vi "YAG_Control.v6.vi"() -> ()   [LabVIEW 2022 SP3]
uses:
  YAGControl.ctl
panel:
  in  "VISA resource name":refnum<visa-resource-name>="BigSky"
  in  "Cluster":T1={"Lamp mode"=TRUE, "Lamps"=FALSE, "Shutter"=FALSE, "Q-Switch"=FALSE, "Int Rep Rate  "=15.0, "Voltage "=700.0, "Temperature"=39.0, "Quit"=FALSE} {"Int Rep Rate" min=1.0 max=30.0; "Temperature" format="%#.0f"; "Voltage" min=680.0 max=990.0 step=1.0}
  in  "Send":bool
  out "Last Response":string
  in  "Other Command":string="vmo1100"
  # "o"
  # "C"
  # "Hz"
  # "V"
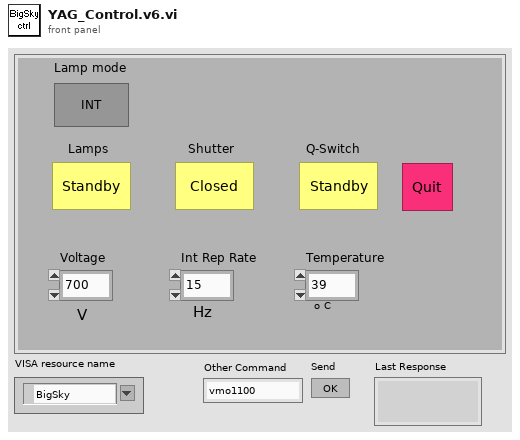
[diagram p1: front panel]
types:
  T1 = typedef "YAGControl.ctl" = cluster{"Lamp mode":bool, "Lamps":bool, "Shutter":bool, "Q-Switch":bool, "Int Rep Rate  ":dbl, "Voltage ":dbl, "Temperature":dbl, "Quit":bool}
  T2 = enum8{"Enabled", "Disabled", "Disabled and Grayed Out"}
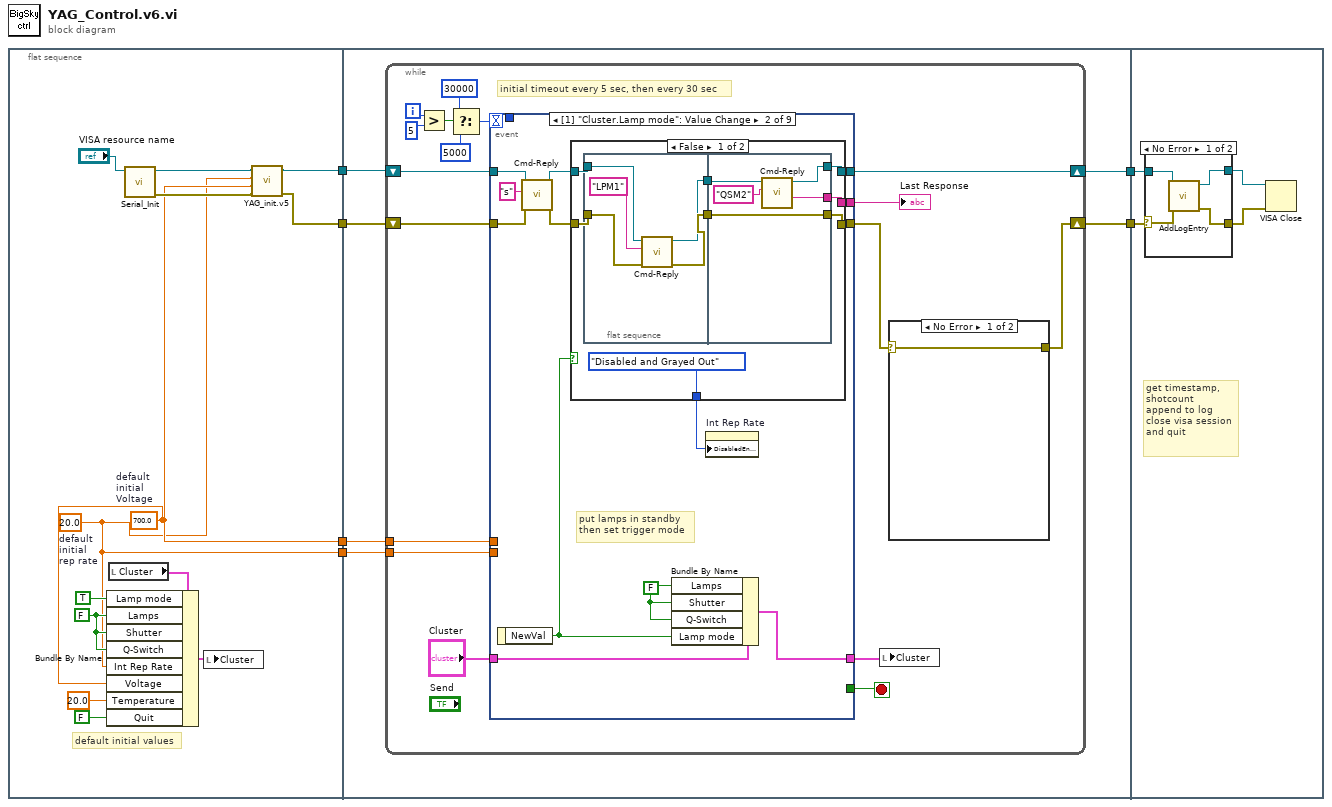
[diagram p0: block diagram]
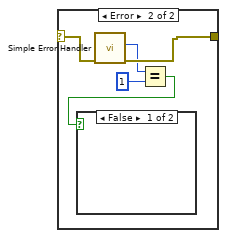
[diagram p2: hidden frame]
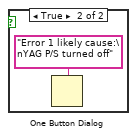
[diagram p3: hidden frame]
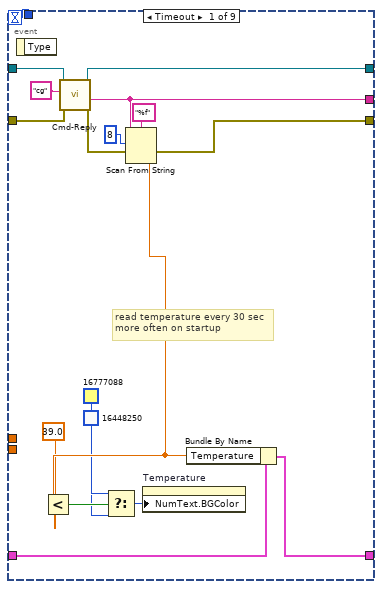
[diagram p4: hidden frame]
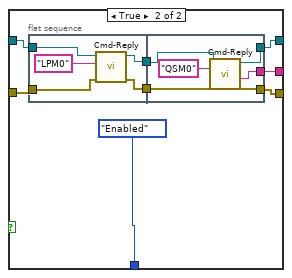
[diagram p5: hidden frame]
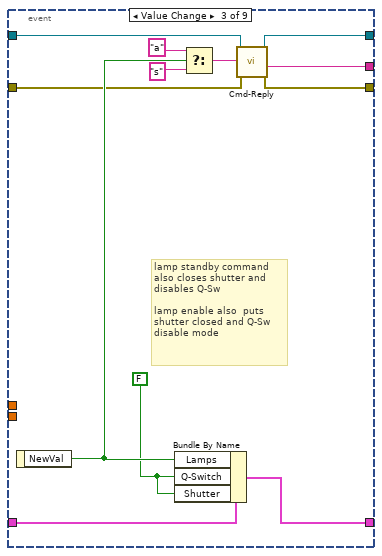
[diagram p6: hidden frame]
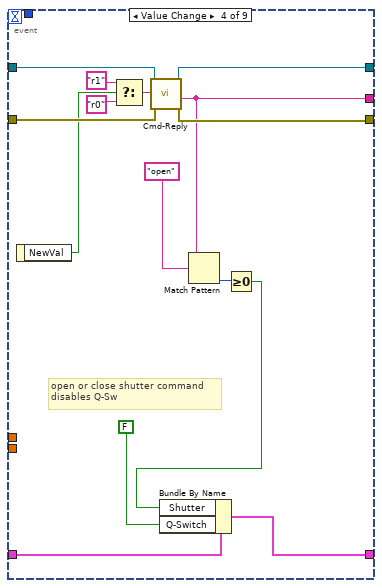
[diagram p7: hidden frame]
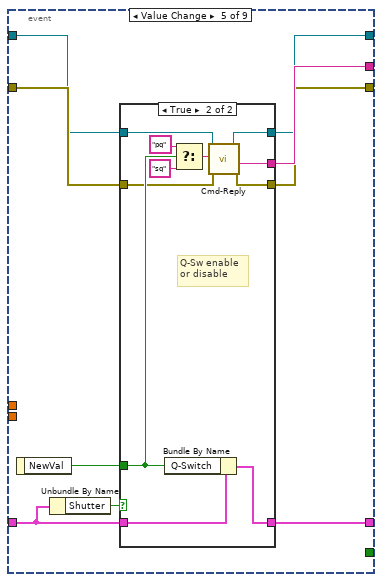
[diagram p8: hidden frame]
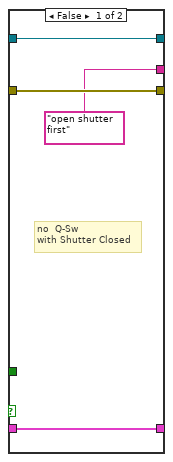
[diagram p9: hidden frame]
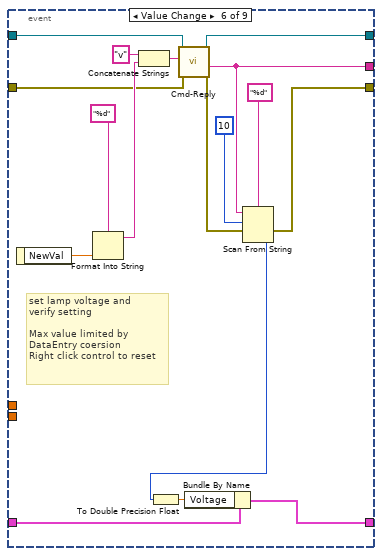
[diagram p10: hidden frame]
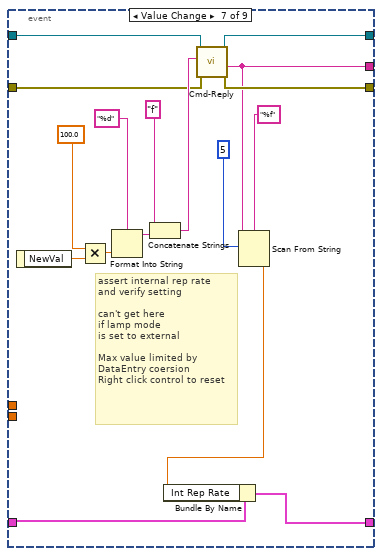
[diagram p11: hidden frame]
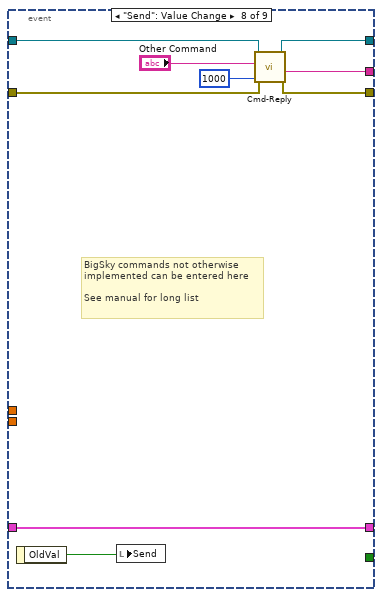
[diagram p12: hidden frame]
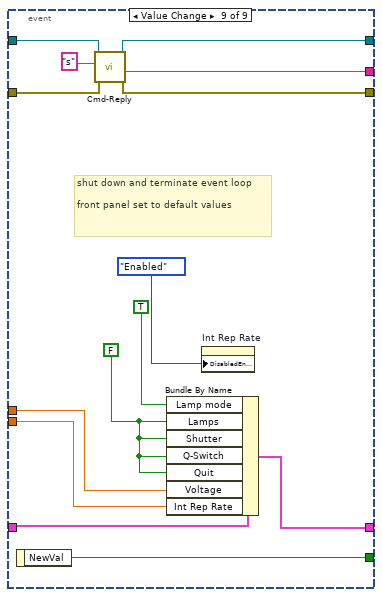
[diagram p13: hidden frame]
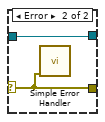
[diagram p14: hidden frame]
diagram:
  n1 = flat-sequence {
    tunnel: [w11] -> w4
    tunnel: [w10] -> w3
    tunnel: [w8] -> w2
    tunnel: [w7] -> w1
    tunnel: [w25] -> w6
    tunnel: [w24] -> w5
    tunnel: w4 -> [w23]
    tunnel: w3 -> [w22]
    tunnel: w2 -> [w21]
    tunnel: w1 -> [w20]
    tunnel: w6 -> [w225]
    tunnel: w5 -> [w228]
    frame #0 {
      w7 = 20.0  # default initial rep rate
      w8 = 700.0  # default  initial Voltage
      w18 = FALSE ("Lamp mode")
      # "default initial values"
      n2 = local read "Cluster"() -> (w13:T1)
      n3 = Bundle By Name(cluster=w13, "Lamp mode"=TRUE, "Lamps"=w18, "Shutter"=w18, "Q-Switch"=w18, "Int Rep Rate"=w7, "Voltage"=w8, "Temperature"=20.0, "Quit"=FALSE) -> (w15:T1)
      n4 = call "Serial_Init.vi"("VISA resource name"="VISA resource name") -> ("error out"=w9:errorcluster, "VISA resource name out"=w12:refnum<visa-resource-name>)  [unwired: 9 in]
      n5 = local write "Cluster"(w15) -> ()
      n6 = call "YAG_init.v5.vi"("error in (no error)"=w9, "initial V"=w8, "initial rep rate"=w7, "VISA Refnum in"=w12) -> ("error out"=w10:errorcluster, "VISA Refnum out"=w11:refnum<visa-resource-name>)  [unwired: 6 in]
    }
    frame #1 {
      n7 = while {
        shift-right: [w36] -> w24
        shift-left: w23 -> [w38]
        shift-right: [w34] -> w25
        shift-left: w22 -> [w37]
        tunnel: w21 -> [w27]
        tunnel: w20 -> [w26]
        i -> [w30]
        stop <- w42 stop-if-true
        # "initial timeout every 5 sec, then every 30 sec"
        n8 = Greater?(x=w30, y=5) -> (0:w28:bool)
        n9 = Select(t=30000, s=w28, f=5000) -> (s? t:f=w33:i32)
        n10 = event shown="[1] \"Cluster.Lamp mode\": Value Change" {
          selector: _ -> [_ _ _ _ _ _ _ _ _]
          dyn-events: _ -> [_ _ _ _ _ _ _ _ _]
          timeout: w33 -> [w51 _ _ _ _ _ _ _ _]
          tunnel: [_ _ _ _ _ _ _ _ w222] -> w42
          tunnel: "Cluster" -> [w67 w80 w128 w143 w150 w168 w200 w210 w224]
          tunnel: [w66 w79 w123 w142 w152 w184 w199 w210 w223] -> w39
          tunnel: [w61 w77 w122 w133 w148 w174 w189 w208 w216] -> w41
          tunnel: w38 -> [w63 w72 w118 w136 w144 w176 w191 w206 w219]
          tunnel: w37 -> [w64 w69 w119 w135 w145 w178 w190 w205 w220]
          tunnel: [w58 w73 w120 w137 w146 w170 w198 w204 w215] -> w35
          tunnel: [w62 w74 w121 w138 w147 w177 w197 w203 w217] -> w36
          tunnel: [w51 _ _ _ _ _ _ _ _] -> _
          tunnel: w27 -> [_ _ _ _ _ _ _ _ w212]
          tunnel: w26 -> [_ _ _ _ _ _ _ _ w211]
          event Timeout {
            # "read temperature every 30 sec\nmore often on startup"
            n11 = event-data() -> ()  [unwired: 1 in, 1 out]
            n12 = call "Cmd-Reply.vi"("error in (no error)"=w64, "cmd"="cg" ("write buffer"), "VISA Refnum in"=w63) -> ("error out"=w59:errorcluster, "reply"=w61:string, "VISA Refnum out"=w62:refnum<visa-resource-name>)  [unwired: 6 in]
            n13 = Scan From String(format string="%f", input string=w61, initial scan location=u32 8, error in=w59) -> (error out=w58:errorcluster, output 1=w57:dbl)  [unwired: 1 in, 2 out]
            n14 = Less?(x=w57, y=39.0) -> (x < y?=w54:bool)
            n15 = Select(t=u32 16777088 ("Color"), s=w54, f=u32 16448250 ("Color")) -> (s? t:f=w55:u32)
            n16 = property on="Temperature" class="DigNum (strict)"("NumText.BGColor"=w55) -> ()  [unwired: 2 in, 2 out]
            n17 = Bundle By Name(cluster=w67, "Temperature"=w57) -> (w66:T1)
          }
          event Value Change {
            w78 = FALSE
            # "put lamps in standby\nthen set trigger mode"
            n18 = event-data() -> ("NewVal"=w75:bool)  [unwired: 1 in]
            n19 = call "Cmd-Reply.vi"("error in (no error)"=w69, "cmd"="s" ("write buffer"), "VISA Refnum in"=w72) -> ("error out"=w68:errorcluster, "VISA Refnum out"=w71:refnum<visa-resource-name>)  [unwired: 6 in, 1 out]
            n20 = case shown="False" w75 {
              tunnel: [w83 w101] -> w77
              tunnel: [T2."Disabled and Grayed Out" ("Disabled") T2."Enabled" ("Disabled")] -> w76
              tunnel: [w87 w104] -> w74
              tunnel: [w86 w102] -> w73
              tunnel: w71 -> [w85 w105]
              tunnel: w68 -> [w84 w103]
              frame False {
                n21 = flat-sequence {
                  tunnel: [w93] -> w82
                  tunnel: w85 -> [w92]
                  tunnel: w84 -> [w91]
                  tunnel: [w89] -> w81
                  tunnel: [w95] -> w87
                  tunnel: [w94] -> w86
                  tunnel: w82 -> [w94]
                  tunnel: [w97] -> w83
                  tunnel: w81 -> [w96]
                  frame #0 {
                    n22 = call "Cmd-Reply.vi"("error in (no error)"=w91, "cmd"="LPM1", "VISA Refnum in"=w92) -> ("error out"=w93:errorcluster, "VISA Refnum out"=w89:refnum<visa-resource-name>)  [unwired: 6 in, 1 out]
                  }
                  frame #1 {
                    n23 = call "Cmd-Reply.vi"("cmd"="QSM2", "VISA Refnum in"=w96) -> ("reply"=w97:string, "VISA Refnum out"=w95:refnum<visa-resource-name>)  [unwired: 7 in, 1 out]
                  }
                }
              }
              frame True {
                n24 = flat-sequence {
                  tunnel: w105 -> [w110]
                  tunnel: w103 -> [w109]
                  tunnel: [w108] -> w100
                  tunnel: [w107] -> w99
                  tunnel: [w114] -> w104
                  tunnel: [w112] -> w102
                  tunnel: w100 -> [w112]
                  tunnel: [w113] -> w101
                  tunnel: w99 -> [w115]
                  frame #0 {
                    n25 = call "Cmd-Reply.vi"("error in (no error)"=w109, "cmd"="LPM0", "VISA Refnum in"=w110) -> ("error out"=w108:errorcluster, "VISA Refnum out"=w107:refnum<visa-resource-name>)  [unwired: 6 in, 1 out]
                  }
                  frame #1 {
                    n26 = call "Cmd-Reply.vi"("cmd"="QSM0", "VISA Refnum in"=w115) -> ("reply"=w113:string, "VISA Refnum out"=w114:refnum<visa-resource-name>)  [unwired: 7 in, 1 out]
                  }
                }
              }
            }
            n27 = Bundle By Name(cluster=w80, "Lamps"=w78, "Shutter"=w78, "Q-Switch"=w78, "Lamp mode"=w75) -> (w79:T1)
            n28 = property on="Int Rep Rate" class="DigNum (strict)"("DisabledEnum"=w76) -> ()  [unwired: 2 in, 2 out]
          }
          event Value Change {
            w124 = FALSE
            # "lamp standby command\nalso closes shutter and\ndisables Q-Sw\n\nlamp enable also  puts\nshutter closed and Q-Sw \ndisable mode"
            n29 = event-data() -> ("NewVal"=w125:bool)  [unwired: 1 in]
            n30 = Bundle By Name(cluster=w128, "Lamps"=w125, "Q-Switch"=w124, "Shutter"=w124) -> (w123:T1)
            n31 = Select(t="a", s=w125, f="s") -> (s? t:f=w117:string)
            n32 = call "Cmd-Reply.vi"("error in (no error)"=w119, "cmd"=w117, "VISA Refnum in"=w118) -> ("error out"=w120:errorcluster, "reply"=w122:string, "VISA Refnum out"=w121:refnum<visa-resource-name>)  [unwired: 6 in]
          }
          event Value Change {
            # "open or close shutter command\ndisables Q-Sw"
            n33 = event-data() -> ("NewVal"=w130:bool)  [unwired: 1 in]
            n34 = Select(t="r1", s=w130, f="r0") -> (s? t:f=w134:string)
            n35 = call "Cmd-Reply.vi"("error in (no error)"=w135, "cmd"=w134, "VISA Refnum in"=w136) -> ("error out"=w137:errorcluster, "reply"=w133:string, "VISA Refnum out"=w138:refnum<visa-resource-name>)  [unwired: 6 in]
            n36 = Match Pattern(string=w133, regular expression="open") -> (offset past match=w131:i32)  [unwired: 1 in, 3 out]
            n37 = Greater Or Equal To 0?(x=w131) -> (x >= 0?=w129:bool)
            n38 = Bundle By Name(cluster=w143, "Shutter"=w129, "Q-Switch"=FALSE) -> (w142:T1)
          }
          event Value Change {
            n39 = event-data() -> ("NewVal"=w151:bool)  [unwired: 1 in]
            n40 = Unbundle By Name(w150) -> ("Shutter"=w149:bool)
            n41 = case shown="True" w149 {
              tunnel: [w156 w163] -> w152
              tunnel: w151 -> [_ w164]
              tunnel: w150 -> [w156 w167]
              tunnel: ["open shutter first" w162] -> w148
              tunnel: [w155 w161] -> w147
              tunnel: [w154 w160] -> w146
              tunnel: w145 -> [w154 w159]
              tunnel: w144 -> [w155 w158]
              frame False {
                # "no  Q-Sw \nwith Shutter Closed"
              }
              frame True {
                # "Q-Sw enable\nor disable"
                n42 = Bundle By Name(cluster=w167, "Q-Switch"=w164) -> (w163:T1)
                n43 = Select(t="pq", s=w164, f="sq") -> (s? t:f=w157:string)
                n44 = call "Cmd-Reply.vi"("error in (no error)"=w159, "cmd"=w157, "VISA Refnum in"=w158) -> ("error out"=w160:errorcluster, "reply"=w162:string, "VISA Refnum out"=w161:refnum<visa-resource-name>)  [unwired: 6 in]
              }
            }
          }
          event Value Change {
            # "set lamp voltage and\nverify setting\n\nMax value limited by\nDataEntry coersion \nRight click control to reset"
            n45 = event-data() -> ("NewVal"=w182:dbl)  [unwired: 1 in]
            n46 = Format Into String(format string="%d", w182) -> (resulting string=w180:string)  [unwired: 2 in, 1 out]
            n47 = Concatenate Strings("v" ("string"), w180) -> (w181:string)
            n48 = call "Cmd-Reply.vi"("error in (no error)"=w178, "cmd"=w181, "VISA Refnum in"=w176) -> ("error out"=w171:errorcluster, "reply"=w174:string, "VISA Refnum out"=w177:refnum<visa-resource-name>)  [unwired: 6 in]
            n49 = Scan From String(format string="%d", input string=w174, initial scan location=u32 10, error in=w171) -> (error out=w170:errorcluster, output 1=w175:i32)  [unwired: 1 in, 2 out]
            n50 = To Double Precision Float(number=w175) -> (double precision float=w169:dbl)
            n51 = Bundle By Name(cluster=w168, "Voltage"=w169) -> (w184:T1)
          }
          event Value Change {
            # "assert internal rep rate\nand verify setting\n\ncan't get here  \nif lamp mode\nis set to external\n\nMax value limited by\nDataEntry coersion \nRight click control to reset"
            n52 = event-data() -> ("NewVal"=w186:dbl)  [unwired: 1 in]
            n53 = Multiply(x=100.0, y=w186) -> (x*y=w194:dbl)
            n54 = Format Into String(format string="%d", w194) -> (resulting string=w192:string)  [unwired: 2 in, 1 out]
            n55 = Concatenate Strings("f" ("string"), w192) -> (w196:string)
            n56 = call "Cmd-Reply.vi"("error in (no error)"=w190, "cmd"=w196, "VISA Refnum in"=w191) -> ("error out"=w198:errorcluster, "reply"=w189:string, "VISA Refnum out"=w197:refnum<visa-resource-name>)  [unwired: 6 in]
            n57 = Scan From String(format string="%f", input string=w189, initial scan location=u32 5) -> (output 1=w185:dbl)  [unwired: 2 in, 3 out]
            n58 = Bundle By Name(cluster=w200, "Int Rep Rate"=w185) -> (w199:T1)
          }
          event "Send": Value Change {
            # "BigSky commands not otherwise\nimplemented can be entered here\n\nSee manual for long list"
            n59 = event-data() -> ("OldVal"=w209:bool)  [unwired: 1 in]
            n60 = local write "Send"(w209) -> ()
            n61 = call "Cmd-Reply.vi"("error in (no error)"=w205, "ms to wait"=u32 1000, "cmd"="Other Command", "VISA Refnum in"=w206) -> ("error out"=w204:errorcluster, "reply"=w208:string, "VISA Refnum out"=w203:refnum<visa-resource-name>)  [unwired: 5 in]
          }
          event Value Change {
            w221 = FALSE
            # "shut down and terminate event loop\n\nfront panel set to default values"
            n62 = event-data() -> ("NewVal"=w222:bool)  [unwired: 1 in]
            n63 = call "Cmd-Reply.vi"("error in (no error)"=w220, "cmd"="s", "VISA Refnum in"=w219) -> ("error out"=w215:errorcluster, "reply"=w216:string, "VISA Refnum out"=w217:refnum<visa-resource-name>)  [unwired: 6 in]
            n64 = Bundle By Name(cluster=w224, "Lamp mode"=TRUE, "Lamps"=w221, "Shutter"=w221, "Q-Switch"=w221, "Quit"=w221, "Voltage"=w212, "Int Rep Rate"=w211) -> (w223:T1)
            n65 = property on="Int Rep Rate" class="DigNum (strict)"("DisabledEnum"=T2."Enabled" ("Disabled")) -> ()  [unwired: 2 in, 2 out]
          }
        }
        "Last Response" <- w41
        n66 = local write "Cluster"(w39) -> ()
        n67 = case shown="No Error" w35 {
          selector: w35 -> [w43 w48]
          tunnel: [w43 w47] -> w34
          frame No Error {
          }
          frame Error {
            n68 = call <vilib>:"Simple Error Handler.vi"("error in (no error)"=w48) -> ("code out"=w46:i32, "error out"=w47:errorcluster)  [unwired: 4 in, 3 out]
            n69 = Equal?(x=w46, y=1) -> (x = y?=w44:bool)
            n70 = case shown="False" w44 {
              frame False {
              }
              frame True {
                n71 = One Button Dialog(message="Error 1 likely cause:\nYAG P/S turned off") -> ()  [unwired: 1 in, 1 out]
              }
            }
          }
        }
      }
    }
    frame #2 {
      # "get timestamp,\nshotcount\nappend to log\nclose visa session\nand quit"
      n72 = case shown="No Error" w225 {
        selector: w225 -> [w229 w233]
        tunnel: w228 -> [w232 w234]
        tunnel: [w231 w233] -> w227
        tunnel: [w230 w234] -> w226
        frame No Error {
          n73 = call "AddLogEntry.vi"("error in"=w229, "VISA Refnum in"=w232) -> ("error out"=w231:errorcluster, "VISA Refnum out"=w230:refnum<visa-resource-name>)  [unwired: 8 in]
        }
        frame Error {
          n74 = call <vilib>:"Simple Error Handler.vi"("error in (no error)"=w233) -> ()  [unwired: 4 in, 5 out]
        }
      }
      n75 = VISA Close(VISA resource name=w226, error in (no error)=w227) -> ()  [unwired: 1 out]
    }
  }
